vi "Rectangular Target - 2013.vi"(3 "Camera Settings":T3={"FPS"=30, "Compression"=30, "Image Size"=enum."320x240"}, 4 "Target Choice":i8(knob) scale=0.0..2.0, 5 "Camera IP Address":string="192.168.0.90", 6 "Camera Image":T1(plugin-control)) -> (0 "Center Target":bool, 1 "Processed Image":T1(plugin-control), 2 "Numeric Target Info":dbl[](array[numeric]))   [LabVIEW 2012]
doc: "This VI demonstrates how to do target processing on a laptop computer. It uses the same MJPG VI as the dashboard, sets a few of the important camera properties that impact processing, and carries out the same processing steps as the RT example also included in this project."
uses:
  <vilib>/Rock Robotics/WPI/Camera/WPI_CameraImageSize.ctl
  <vilib>/Rock Robotics/WPI/Camera/WPI_CameraWhite Balance Values.ctl
  <vilib>/vision/NI_Vision_Development_Module.lvlib
panel:
  in  "Camera Type":enum16{"206", "1011"}(ring)=enum."1011"
  in  "Image Source":enum32{"Live Camera", "File Images"}(tab)
  in  "Directory":path
  in  "File List":i32(listbox)
  out "Target Info":T4(array[cluster])
  in  "Area Size Limit %":dbl=0.5
  in  "Particle Count Limit":i32=10
  in  "Score Limits":T5={"Rect Coverage"=60.0, "X Edge Strength"=40.0, "Y Edge Strength"=60.0, "Center"=75.0, "Outer"=75.0}
  in  "Processing":enum32{"Color", "Monochrome"}(tab)
  out "Value":cluster{i32, i32}
  out "Saturation":cluster{i32, i32}
  in  "Value":i32=255
  in  "Saturation":i32=255
  in  "Hue":i32(knob)=65 scale=0.0..255.0
  in  "Margins":cluster{"Hue":i32, "Sat":i32, "Val":i32}={"Hue"=33, "Sat"=53, "Val"=9} {"Sat" scale=0.0..80.0; "Val" scale=0.0..80.0; "Hue" scale=0.0..80.0}
  out "Hue":cluster{i32, i32}
  in  "Range":cluster{"Lower value":sgl, "Upper value":sgl}={"Lower value"=150.0, "Upper value"=255.0} {"Lower value" scale=0.0..255.0; "Upper value" scale=0.0..255.0}
  in  "Color Plane":i32(ring)=6 items=["Red", "Green", "Blue", "Hue", "Saturation", "Luminance", "Value", "Intensity"]
  in  "Annotate":bool=TRUE
  out "Original Image":T1(plugin-control)
  # "Information:\nProcessing can be based on color or light intensity.\nParticles within the image are scored by rectangle coverage, aspect ratio, and\nedge strength/hollowness. A particle is considered a target if all scores\nare above the score limits you set. Particles can be annotated -- surrounded by\na rectangle and scores drawn to the left .\nTo control the number of particles being scored, use the count limit and the size\nlimit.\nBe sure to set the Camera IP before running. The distance calculation uses the\ncamera type to index the value of the lens view angle."
  # "Click in the image to choose  color for processing."
  # "Green scores are above the limit, orange are below. Inner/outer rect\nindicates all passed."
  # "Set before running."
  # "Lower/Upper"
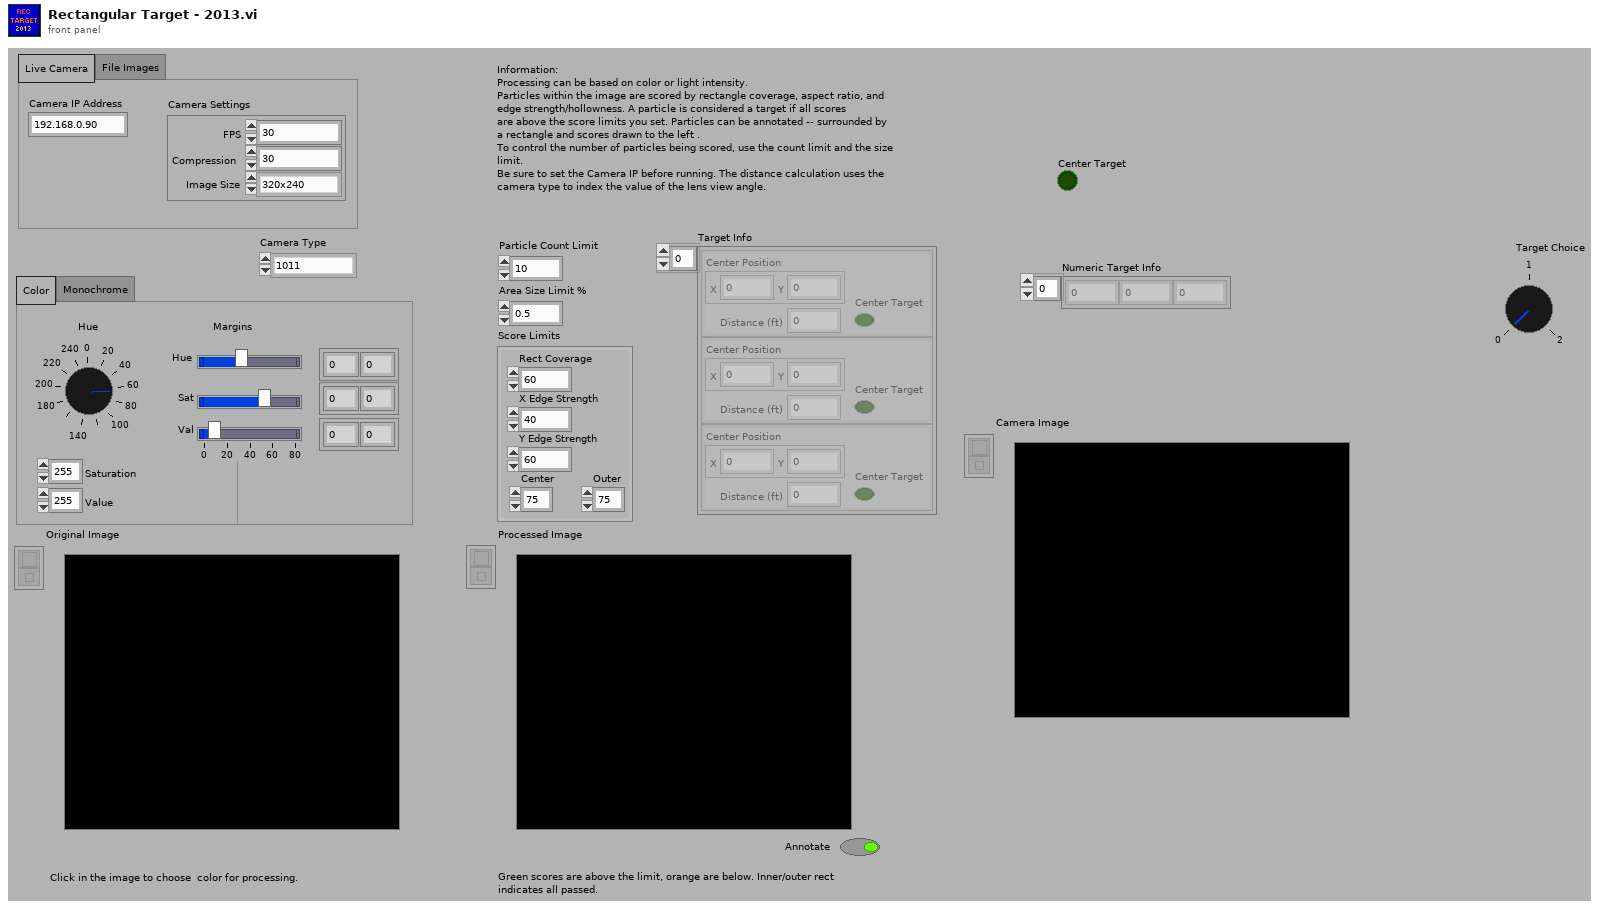
[diagram p1: front panel]
types:
  T1 = typedef "IMAQ Image.ctl" = refnum<image>
  T2 = typedef "WPI_CameraImageSize.ctl" = enum16{"640x480", "320x240", "160x120"}
  T3 = cluster{"FPS":i32, "Compression":i32, "Image Size":T2}
  T4 = cluster{"Center Position":cluster{"X":dbl, "Y":dbl}, "Distance (ft)":dbl, "Center Target":bool}[]
  T5 = cluster{"Rect Coverage":dbl, "X Edge Strength":dbl, "Y Edge Strength":dbl, "Center":dbl, "Outer":dbl}
  T6 = typedef "WPI_CameraWhite Balance Values.ctl" = enum16{"Auto", "Fixed indoor", "Fixed outdoor 1", "Fixed outdoor 2", "Fixed fluorescent 1", "Fixed fluorescent 2", "Hold current"}
  T7 = typedef "Image Type" = u32
  T8 = typedef "WPI_CameraDevRef.ctl" = cluster{"Camera Address":string, "CameraStatus":errorcluster, "Acquire Image Notifier":refnum<notifier>}
  T9 = cluster{"Position":cluster{"X":dbl, "Y":dbl}, "Distance (ft)":dbl, "Center Target":bool}[]
  T10 = cluster{cluster{"Left":dbl, "Top":dbl, "Right":dbl, "Bottom":dbl}, "Scores":dbl[], cluster{"Long":dbl, "Short":dbl}}[]
  T11 = cluster{"Target Center (-1 to 1)":cluster{"X":dbl, "Y":dbl}, "Distance (ft)":dbl, "Center Target":bool}
  T12 = cluster{"Target Center (-1 to 1)":cluster{"X":dbl, "Y":dbl}, "Distance (ft)":dbl, "Center Target":bool}[]
  T13 = cluster{"Left":dbl, "Top":dbl, "Right":dbl, "Bottom":dbl}
  T14 = cluster{"Position":cluster{"X":dbl, "Y":dbl}, "Distance (ft)":dbl, "Center Target":bool}
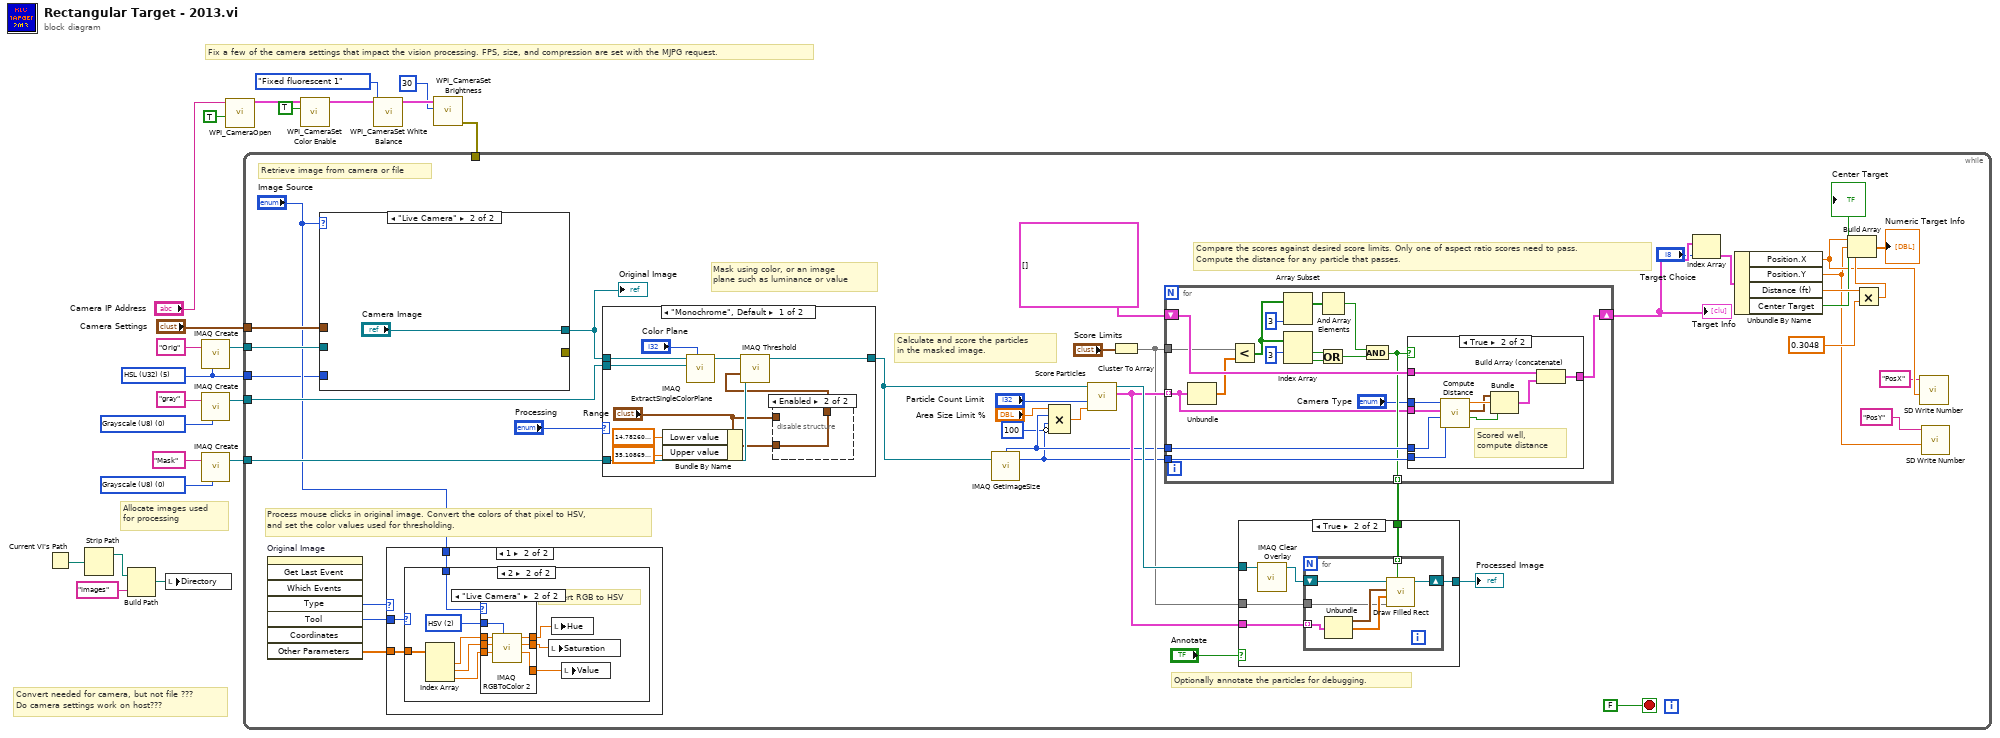
[diagram p0: block diagram]
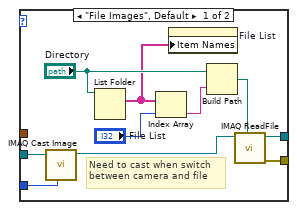
[diagram p2: hidden frame]
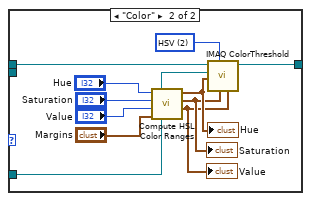
[diagram p5: hidden frame]
diagram:
  w17 = T7 0 items=["Grayscale (U8)", "Grayscale (I16)", "Grayscale (SGL)", "Complex (CSG)", "RGB (U32)", "HSL (U32)", "RGB (U64)", "Grayscale (U16)"] ("Image Type")
  w2 = T7 5 items=["Grayscale (U8)", "Grayscale (I16)", "Grayscale (SGL)", "Complex (CSG)", "RGB (U32)", "HSL (U32)", "RGB (U64)", "Grayscale (U16)"] ("Image Type")
  w23 = T7 0 items=["Grayscale (U8)", "Grayscale (I16)", "Grayscale (SGL)", "Complex (CSG)", "RGB (U32)", "HSL (U32)", "RGB (U64)", "Grayscale (U16)"] ("Image Type")
  # "Convert needed for camera, but not file ???\nDo camera settings work on host???"
  # "Allocate images used\nfor processing"
  # "Fix a few of the camera settings that impact the vision processing. FPS, size, and compression are set with the MJPG request."
  n1 = Current VI's Path() -> (path=w6:path)
  n2 = Strip Path(path=w6) -> (stripped path=w4:path)  [unwired: 1 out]
  n3 = Build Path(base path=w4, name or relative path="images") -> (appended path=w3:path)
  n4 = local write "Directory"(w3) -> ()
  n5 = call "IMAQ Create"("Image Name"="Orig", "Image Type"=w2) -> ("New Image"=w20:T1)  [unwired: 2 in, 2 out]
  n6 = call "IMAQ Create"("Image Name"="gray", "Image Type"=w23) -> ("New Image"=w19:T1)  [unwired: 2 in, 2 out]
  n7 = call "IMAQ Create"("Image Name"="Mask", "Image Type"=w17) -> ("New Image"=w16:T1)  [unwired: 2 in, 2 out]
  n8 = call <vilib>:"WPI_CameraOpen.vi"("Disallow Simulation"=TRUE, "Camera Address"="Camera IP Address") -> ("CameraDevRef"=w12:T8)  [unwired: 8 in, 1 out]
  n9 = call <vilib>:"WPI_CameraSet Color Enable.vi"("Color Enabled"=TRUE, "CameraDevRef"=w12) -> ("CameraDevRef Out"=w10:T8)  [unwired: 8 in, 1 out]
  n10 = call <vilib>:"WPI_CameraSet White Balance.vi"("White Balance"=WPI_CameraWhite_Balance_Values."Fixed fluorescent 1", "CameraDevRef"=w10) -> ("CameraDevRef Out"=w8:T8)  [unwired: 8 in, 1 out]
  n11 = call <vilib>:"WPI_CameraSet Brightness.vi"("Brightness"=30, "CameraDevRef"=w8) -> ("error out"=w14:errorcluster)  [unwired: 8 in, 1 out]
  n12 = while {
    tunnel: w20 -> [w56]
    tunnel: w19 -> [w62]
    tunnel: w16 -> [w43]
    tunnel: w14 -> [_]
    tunnel: "Camera Settings" -> [w46]
    tunnel: w2 -> [w41]
    stop <- FALSE stop-if-true
    # "Retrieve image from camera or file"
    # "Optionally annotate the particles for debugging."
    # "Compare the scores against desired score limits. Only one of aspect ratio scores need to pass.\nCompute the distance for any particle that passes."
    # "Process mouse clicks in original image. Convert the colors of that pixel to HSV,\nand set the color values used for thresholding."
    # "Calculate and score the particles\nin the masked image."
    # "Mask using color, or an image\nplane such as luminance or value"
    n13 = invoke on="Original Image" class="ImageControl" method="Get Last Event"() -> ("Type"=w57:i32, "Tool"=w58:i32, "Other Parameters"=w59:sgl[])  [unwired: 8 in, 5 out]
    n14 = case shown="\"Live Camera\"" "Image Source" {
      tunnel: w56 -> [w65 _]
      tunnel: [w72 "Camera Image"] -> w55
      tunnel: w46 -> [_ _]
      tunnel: [w71 _] -> _
      tunnel: w41 -> [w63 _]
      frame "File Images", Default {
        # "Need to cast when switch\nbetween camera and file"
        n15 = call "IMAQ Cast Image"("Image Type"=w63, "Image Src"=w65) -> ("Image Dst Out"=w64:T1)  [unwired: 8 in, 1 out]
        n16 = List Folder(path="Directory") -> (filenames=w66:string[])  [unwired: 3 in, 3 out]
        n17 = Index Array(array=w66, index="File List") -> (element=w69:string)
        n18 = property on="File List" class="LstBox (strict)"("Item Names"=w66) -> ()  [unwired: 2 in, 2 out]
        n19 = Build Path(base path="Directory", name or relative path=w69) -> (appended path=w68:path)
        n20 = call "IMAQ ReadFile"("File Path"=w68, "Image"=w64) -> ("error out"=w71:errorcluster, "Image Out"=w72:T1)  [unwired: 5 in, 3 out]
      }
      frame "Live Camera" {
      }
    }
    "Original Image" <- w55
    n21 = case shown="1" w57 {
      tunnel: w58 -> [_ w142]
      tunnel: w59 -> [_ w141]
      tunnel: "Image Source" -> [_ w140]
      frame 0, Default {
      }
      frame 1 {
        n22 = case shown="2" w142 {
          tunnel: w141 -> [_ w151]
          tunnel: w140 -> [_ w143]
          frame Default {
          }
          frame 2 {
            w150 = u16 2 items=["RGB", "HSL", "HSV", "HSI", "CIE L*a*b*", "CIE XYZ"] ("Color Mode")
            # "Convert RGB to HSV"
            n23 = Index Array(array=w151) -> (element #1=w149:sgl, element #2=w147:sgl, element #3=w145:sgl)  [unwired: 3 in]
            n24 = case shown="\"Live Camera\"" w143 {
              tunnel: w150 -> [_ w161]
              tunnel: w149 -> [w154 w160]
              tunnel: [w154 w159] -> w148
              tunnel: w147 -> [w153 w158]
              tunnel: [w153 w157] -> w146
              tunnel: w145 -> [w152 w156]
              tunnel: [w152 w155] -> w144
              frame "File Images", Default {
              }
              frame "Live Camera" {
                n25 = call "IMAQ RGBToColor 2"("Color Mode"=w161, "Blue value"=w156, "Green value"=w158, "Red value"=w160) -> ("Blue or Luma or Val or Inten or Z or b*value"=w155:dbl, "Green or Sat or Y or a* value"=w157:dbl, "Red or Hue or X or L* value"=w159:dbl)  [unwired: 4 in, 1 out]
              }
            }
            n26 = local write "Saturation"(w146) -> ()
            n27 = local write "Hue"(w148) -> ()
            n28 = local write "Value"(w144) -> ()
          }
        }
      }
    }
    n29 = case shown="\"Monochrome\", Default" "Processing" {
      tunnel: w55 -> [w98 w111]
      tunnel: w62 -> [w97 _]
      tunnel: [w95 w110] -> w49
      tunnel: w43 -> [w93 w101]
      frame "Monochrome", Default {
        n30 = Bundle By Name(cluster="Range", "Lower value"=sgl 14.7826, "Upper value"=sgl 35.1087) -> (w89:cluster{"Lower value":sgl, "Upper value":sgl})
        n31 = call "IMAQ ExtractSingleColorPlane"("Color Plane"="Color Plane", "Image Dst"=w97, "Image Src"=w98) -> ("Image Dst Out"=w96:T1)  [unwired: 1 in, 7 out]
        n32 = disable-structure shown="Enabled" {
          disable-tunnel: [w99 w100] -> w90
          disable-tunnel: w89 -> [_ w100]
          disable-tunnel: "Range" -> [w99 _]
          frame Disabled {
          }
          frame Enabled {
          }
        }
        n33 = call "IMAQ Threshold"("Range"=w90, "Image Dst"=w93, "Image Src"=w96) -> ("Image Dst Out"=w95:T1)  [unwired: 3 in, 5 out]
      }
      frame "Color" {
        w109 = u16 2 items=["RGB", "HSL", "HSV", "HSI"] ("Color Mode")
        n34 = call "Compute HSL Color Ranges.vi"("Margins"="Margins", "Luminance"="Value", "Saturation"="Saturation", "Hue"="Hue") -> ("Lum Range"=w102:cluster{i32, i32}, "Sat Range"=w103:cluster{i32, i32}, "Hue Range"=w108:cluster{i32, i32})  [unwired: 5 in]
        "Hue" <- w108
        "Saturation" <- w103
        "Value" <- w102
        n35 = call "IMAQ ColorThreshold"("Blue or Luma or Val or Inten Range"=w102, "Green or Sat Range"=w103, "Color Mode"=w109, "Red or Hue Range"=w108, "Image Dst"=w101, "Image Src"=w111) -> ("Image Dst Out"=w110:T1)  [unwired: 4 in, 1 out]
      }
    }
    n36 = call "IMAQ GetImageSize"("Image"=w49) -> ("Y Resolution"=w38:i32, "X Resolution"=w39:i32)  [unwired: 3 in, 1 out]
    n37 = Compound Arithmetic op=MULTIPLY("Area Size Limit %", w39, w38, invert 100 ("value")) -> (w37:dbl)
    n38 = call "Score Particles.vi"("Area Size Limit"=w37, "Particle Count Limit"="Particle Count Limit", "Image Refnum in"=w49) -> ("Scored Particle Info"=w51:T10, "Image Refnum out"=w54:T1)  [unwired: 7 in]
    n39 = Cluster To Array(cluster="Score Limits") -> (array=w45:dbl[])
    n40 = for {
      shift-right: [w127] -> w35
      shift-left: T9 [] -> [w128]
      tunnel: w39 -> [w126]
      tunnel: w51 -> [w112] mode=indexing
      tunnel: w45 -> [w124]
      tunnel: w38 -> [w123]
      tunnel: [w114] -> w44 mode=indexing
      n41 = Unbundle(w112) -> ("Scores"=w125:dbl[])  [unwired: 2 out]
      n42 = Less?(x=w124, y=w125) -> (x < y?=w120:bool[])
      n43 = Array Subset(array=w120, length=3) -> (w121:bool[])  [unwired: 1 in]
      n44 = Index Array(array=w120, index #1=3 ("length")) -> (element #1=w118:bool, element #2=w117:bool)  [unwired: 1 in]
      n45 = And Array Elements(Boolean array=w121) -> (logical AND=w115:bool)
      n46 = Or(x=w118, y=w117) -> (x .or. y?=w116:bool)
      n47 = And(x=w115, y=w116) -> (x .and. y?=w114:bool)
      n48 = case shown="True" w114 {
        tunnel: w128 -> [w129 w139]
        tunnel: [w129 w138] -> w127
        tunnel: w126 -> [_ w136]
        tunnel: "Camera Type" -> [_ w134]
        tunnel: w123 -> [_ w132]
        tunnel: w112 -> [_ w131]
        frame False {
          # "Didn't score well enough"
        }
        frame True {
          # "Scored well,\ncompute distance"
          n49 = call "Compute Distance.vi"("Y Image Resolution"=w132, "X Image Resolution"=w136, "Particle Scores"=w131, "Camera Type"=w134) -> ("Center Target"=w130:bool, "Target Center (-1 to 1)"=w133:cluster{"X":dbl, "Y":dbl}, "Distance (ft)"=w135:dbl)  [unwired: 5 in]
          n50 = Bundle("Target Center (-1 to 1)"=w133, "Distance (ft)"=w135, "Center Target"=w130) -> (w137:T11)  [unwired: 1 in]
          n51 = Build Array (concatenate)(w139, w137) -> (w138:T12)
        }
      }
    }
    "Target Info" <- w35
    n52 = case shown="True" "Annotate" {
      tunnel: w54 -> [w74 w80]
      tunnel: [w74 w79] -> w52
      tunnel: w51 -> [_ w77]
      tunnel: w45 -> [_ w76]
      tunnel: w44 -> [_ w75]
      frame False {
      }
      frame True {
        n53 = call "IMAQ Clear Overlay"("Image"=w80) -> ("Image Out"=w78:T1)  [unwired: 2 in, 8 out]
        n54 = for {
          shift-right: [w86] -> w79
          shift-left: w78 -> [w87]
          tunnel: w77 -> [w83] mode=indexing
          tunnel: w76 -> [w82]
          tunnel: w75 -> [w81] mode=indexing
          n55 = Unbundle(w83) -> (w84:T13, "Scores"=w85:dbl[])  [unwired: 1 out]
          n56 = call "Draw Filled Rect.vi"("Limit Passed"=w81, "Limits"=w82, "Scores"=w85, "Bounding Box"=w84, "image in"=w87) -> ("image out"=w86:T1)  [unwired: 6 in]
        }
      }
    }
    "Processed Image" <- w52
    n57 = Index Array(array=w35, index="Target Choice") -> (element=w33:T14)
    n58 = Unbundle By Name(w33) -> ("Position.X"=w27:dbl, "Position.Y"=w26:dbl, "Distance (ft)"=w32:dbl, "Center Target"=→"Center Target":bool)
    n59 = Multiply(x=w32, y=0.3048) -> (x*y=w30:dbl)
    n60 = Build Array(w27, w26, w30) -> (→"Numeric Target Info":dbl[])
    n61 = call <vilib>:"SD Write Number.vi"("Numeric"=w27, "Name"="PosX") -> ()  [unwired: 8 in, 2 out]
    n62 = call <vilib>:"SD Write Number.vi"("Numeric"=w26, "Name"="PosY") -> ()  [unwired: 8 in, 2 out]
  }
